vi "ConvertToErrorUX.vi"(8 "error in (no error)":errorcluster, 11 "ErrorUX":T1) -> (0 "error out":errorcluster)   [LabVIEW 2019, in "LabErrorUX.lvclass"]
uses:
  LabErrorUX.lvclass
  LabErrorUX.lvclass/LabErrorUX.ctl
  Typedefs/ErrorUX.ctl
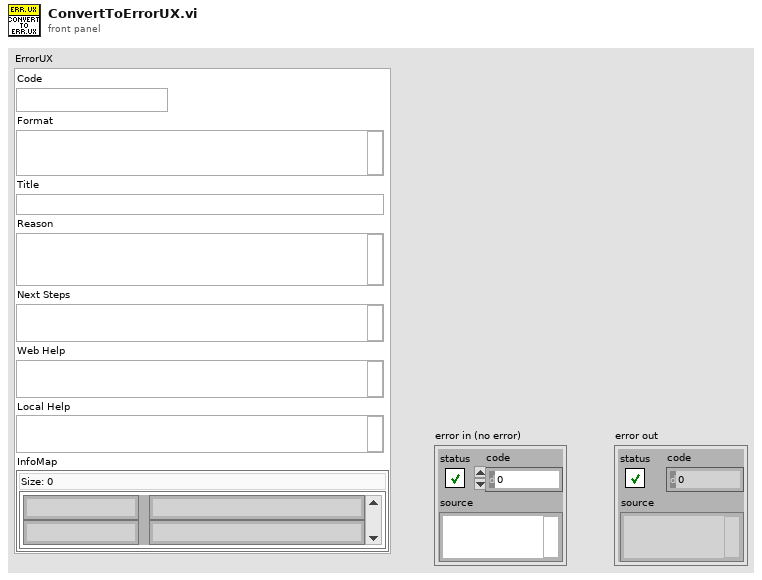
[diagram p1: front panel]
types:
  T1 = typedef "LabErrorUX.lvclass/ErrorUX.ctl" = cluster{"Code":string, "Format":string, "Title":string, "Reason":string, "Next Steps":string, "Web Help":string, "Local Help":string, "InfoMap":map{string, string}}
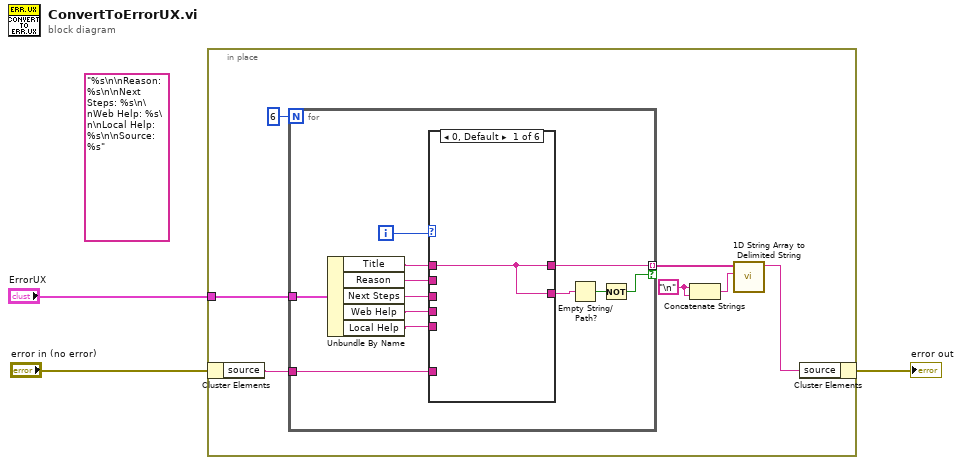
[diagram p0: block diagram]
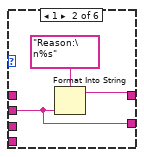
[diagram p2: hidden frame]
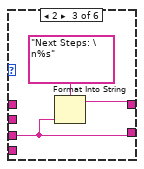
[diagram p3: hidden frame]
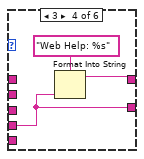
[diagram p4: hidden frame]
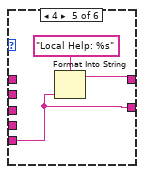
[diagram p5: hidden frame]
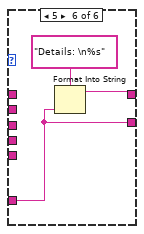
[diagram p6: hidden frame]
diagram:
  (unwired) "%s\n\nReason: %s\n\nNext Steps: %s\n\nWeb Help: %s\n\nLocal Help: %s\n\nSource: %s" ("format string")
  n1 = in-place {
    in-place-border: "ErrorUX" -> [w10]
    w5 = "\n"
    n2 = in-place-cluster #1("error in (no error)") -> ("source"=w9:string)
    n3 = for {
      N: 6 -> [_]
      tunnel: w10 -> [w22]
      tunnel: [w18] -> w8 mode=indexing if=w17
      tunnel: w9 -> [w12]
      i -> [w21]
      n4 = Unbundle By Name(w22) -> ("Title"=w20:string, "Reason"=w16:string, "Next Steps"=w15:string, "Web Help"=w14:string, "Local Help"=w13:string)
      n5 = case shown="0, Default" w21 {
        tunnel: [w23 w25 w28 w31 w34 w37] -> w18
        tunnel: w20 -> [w23 _ _ _ _ _]
        tunnel: w16 -> [_ w24 _ _ _ _]
        tunnel: w15 -> [_ _ w27 _ _ _]
        tunnel: w14 -> [_ _ _ w30 _ _]
        tunnel: w13 -> [_ _ _ _ w33 _]
        tunnel: w12 -> [_ _ _ _ _ w36]
        tunnel: [w23 w24 w27 w30 w33 w36] -> w11
        frame 0, Default {
        }
        frame 1 {
          n6 = Format Into String(format string="Reason:\n%s", w24) -> (resulting string=w25:string)  [unwired: 2 in, 1 out]
        }
        frame 2 {
          n7 = Format Into String(format string="Next Steps: \n%s", w27) -> (resulting string=w28:string)  [unwired: 2 in, 1 out]
        }
        frame 3 {
          n8 = Format Into String(format string="Web Help: %s", w30) -> (resulting string=w31:string)  [unwired: 2 in, 1 out]
        }
        frame 4 {
          n9 = Format Into String(format string="Local Help: %s", w33) -> (resulting string=w34:string)  [unwired: 2 in, 1 out]
        }
        frame 5 {
          n10 = Format Into String(format string="Details: \n%s", w36) -> (resulting string=w37:string)  [unwired: 2 in, 1 out]
        }
      }
      n11 = Empty String/Path?(string/path=w11) -> (empty?=w19:bool)
      n12 = Not(x=w19) -> (.not. x?=w17:bool)
    }
    n13 = Concatenate Strings(w5, w5) -> (w4:string)
    n14 = call <vilib>:"1D String Array to Delimited String.vi"("delimiter"=w4, "string array"=w8) -> ("delimited string"=w7:string)  [unwired: 9 in]
    n15 = in-place-cluster #1("source"=w7) -> (→"error out":errorcluster)
  }
